vi "Get Class Attributes.vi"(8 "error in (no error)":errorcluster, 11 "Setter Generator In":refnum<class "Setter Generator.lvclass">) -> (0 "error out":errorcluster, 3 "Setter Generator Out":refnum<class "Setter Generator.lvclass">)   [LabVIEW 2020, in "Method Generation.lvlib" / "Setter Generator.lvclass"]
uses:
  Setter Generator.lvclass
  Setter Generator.lvclass/Setter Generator.ctl
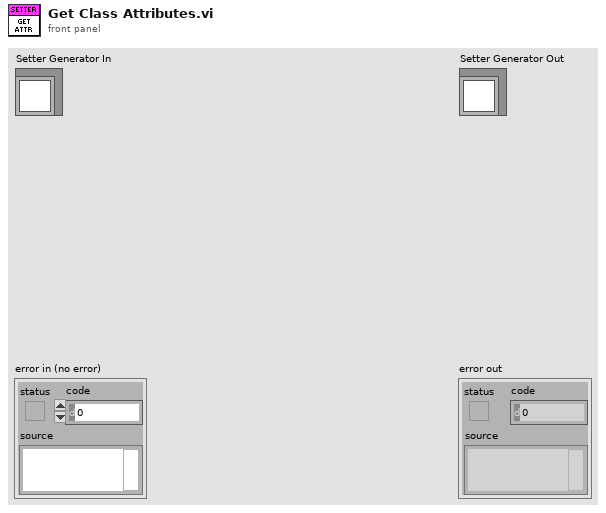
[diagram p1: front panel]
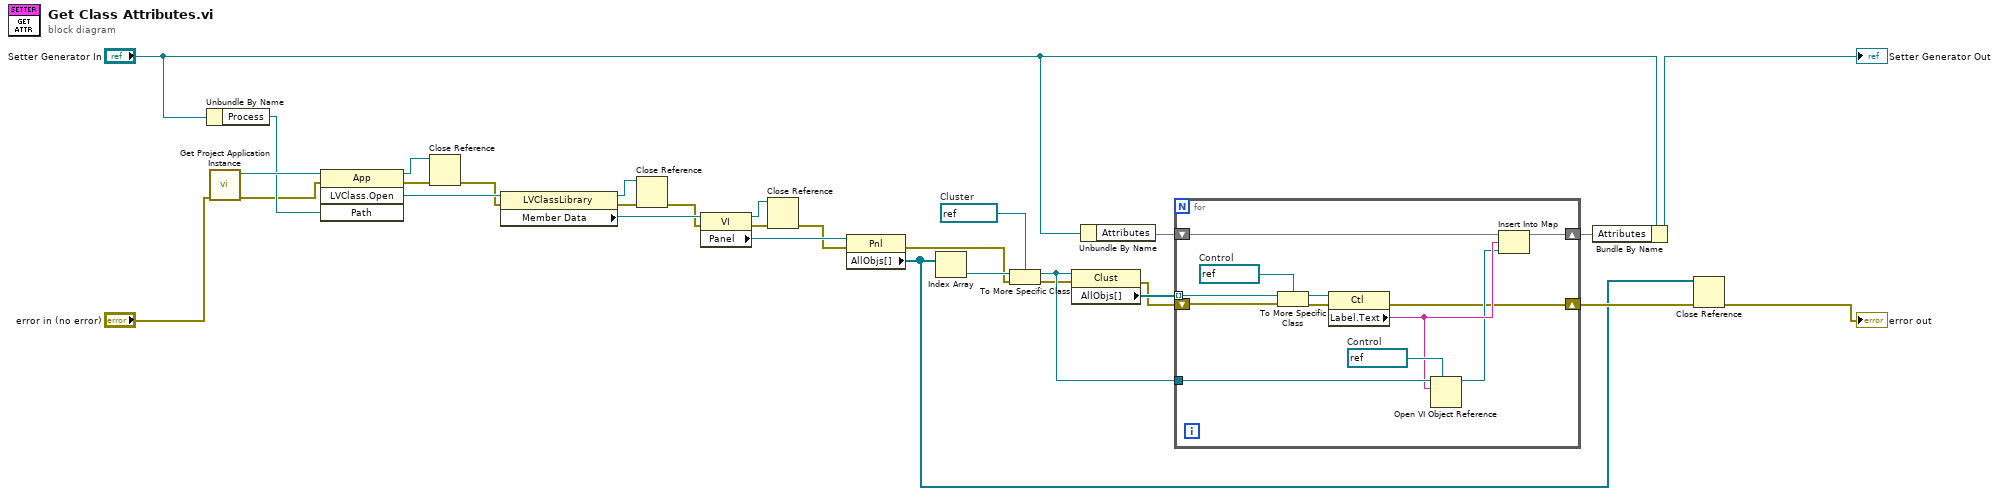
[diagram p0: block diagram]
diagram:
  w22 = refnum<vi> refnum  # Cluster
  n1 = Unbundle By Name("Setter Generator In") -> ("Process"=w29:path)
  n2 = call "Get Project Application Instance.vi"("error in (no error)"="error in (no error)") -> ("error out"=w28:errorcluster, "Application out"=w30:refnum<vi>)  [unwired: 9 in]
  n3 = invoke class="App" method="LVClass.Open"(reference=w30, error in=w28, "Path"=w29) -> (reference out=w7:refnum<vi>, error out=w9:errorcluster, "LVClass.Open"=w26:refnum<vi>)  [unwired: 1 in, 1 out]
  n4 = Close Reference(reference=w7, error in (no error)=w9) -> (error out=w8:errorcluster)
  n5 = property class="LVClassLibrary"(reference=w26, error in=w8) -> (reference out=w5:refnum<vi>, error out=w10:errorcluster, "Member Data"=w25:refnum<vi>)
  n6 = Close Reference(reference=w5, error in (no error)=w10) -> (error out=w6:errorcluster)
  n7 = property class="VI"(reference=w25, error in=w6) -> (reference out=w3:refnum<vi>, error out=w11:errorcluster, "Panel"=w24:refnum<vi>)
  n8 = Close Reference(reference=w3, error in (no error)=w11) -> (error out=w4:errorcluster)
  n9 = property class="Pnl"(reference=w24, error in=w4) -> (error out=w12:errorcluster, "AllObjs[]"=w1:refnum<vi>[])  [unwired: 1 out]
  n10 = Index Array(array=w1) -> (element=w23:refnum<vi>)  [unwired: 1 in]
  n11 = To More Specific Class(target class=w22, reference=w23, error in=w12) -> (specific class reference=w20:refnum<vi>, error out=w13:errorcluster)
  n12 = property class="Clust"(reference=w20, error in=w13) -> (error out=w14:errorcluster, "AllObjs[]"=w21:refnum<vi>[])  [unwired: 1 out]
  n13 = Unbundle By Name("Setter Generator In") -> ("Attributes"=w18:map{string, refnum<vi>})
  n14 = for {
    tunnel: w21 -> [w42] mode=indexing
    tunnel: w20 -> [w39]
    shift-right: [w34] -> w16
    shift-left: w18 -> [w35]
    shift-right: [w33] -> w15
    shift-left: w14 -> [w31]
    w38 = refnum<vi> refnum  # Control
    w40 = refnum<vi> refnum  # Control
    n15 = To More Specific Class(target class=w40, reference=w42, error in=w31) -> (specific class reference=w41:refnum<vi>, error out=w32:errorcluster)
    n16 = property class="Ctl"(reference=w41, error in=w32) -> (error out=w33:errorcluster, "Label.Text"=w37:string)  [unwired: 1 out]
    n17 = Open VI Object Reference(7:w38, 10:w37, 11:w39) -> (3:w36:refnum<vi>)  [unwired: 1 in, 1 out]
    n18 = Insert Into Map(map in=w35, key=w37, value=w36) -> (map out=w34:map{string, refnum<vi>})  [unwired: 2 out]
  }
  n19 = Bundle By Name(cluster="Setter Generator In", "Attributes"=w16) -> (→"Setter Generator Out":refnum<class "Setter Generator.lvclass">)
  n20 = Close Reference(reference=w1, error in (no error)=w15) -> (error out=→"error out":errorcluster)
